vi "Move To Nearest Index.vi"(4 "error in (no error)":errorcluster, 5 "Move Direction (+)":bool=TRUE, 6 "Axis (1)":i32=1 min=1 max=3, 7 "VISA resource name":refnum<visa-resource-name>) -> (0 "error out":errorcluster, 3 "VISA resource name out":refnum<visa-resource-name>)   [LabVIEW 2019, in "Newport ESP301.lvlib"]
doc: "This command is used to move an axis to its nearest index (positive or negative). It uses the home search speed during travel to nearest index.\n<B>NOTE:</B> This command cannot be issued after enabling DAQ (refer ASCII command, DE)."
uses:
  Newport ESP301.lvlib
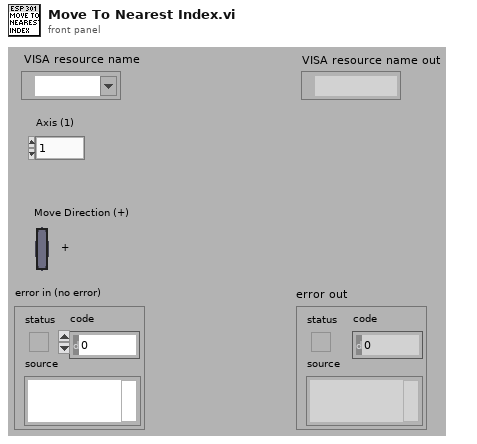
[diagram p1: front panel]
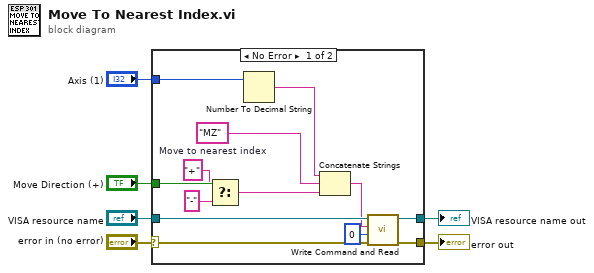
[diagram p0: block diagram]
diagram:
  n1 = case shown="No Error" "error in (no error)" {
    selector: "error in (no error)" -> [w18 w21]
    tunnel: [w17 w21] -> w6
    tunnel: "VISA resource name" -> [w19 w20]
    tunnel: [w16 w20] -> w5
    tunnel: "Axis (1)" -> [w13 _]
    tunnel: "Move Direction (+)" -> [w10 _]
    frame No Error {
      w14 = "MZ"  # Move to nearest index
      n2 = Select(t="+", s=w10, f="-") -> (s? t:f=w7:string)
      n3 = Number To Decimal String(number=w13) -> (decimal integer string=w15:string)  [unwired: 1 out]
      n4 = Concatenate Strings(w15, w14, w7) -> (w12:string)
      n5 = call "Write Command and Read.vi"("error in (no error)"=w18, "Bytes to read (100)"=u32 0, "Command"=w12, "VISA resource name"=w19) -> ("error out"=w17:errorcluster, "VISA resource name out"=w16:refnum<visa-resource-name>)  [unwired: 1 in, 3 out]
    }
    frame Error {
    }
  }
  "error out" <- w6
  "VISA resource name out" <- w5
